vi "G#Debugger_AddObjectToTree.vi"(0 "Front Panel":refnum<vi>, 1 "Tree":refnum<vi>, 2 "Elements":T1[](array[typedef]), 5 "error in (no error)":errorcluster) -> (19 "error out":errorcluster)   [LabVIEW 2017, in "G#Debugger.lvlib"]
uses:
  G#Debugger.lvlib
  G#Debugger_TreeElement.ctl
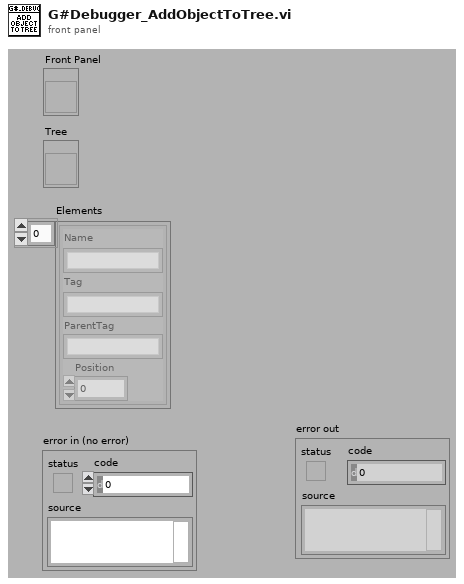
[diagram p1: front panel]
types:
  T1 = typedef "G#Debugger.lvlib/G#Debugger_TreeElement.ctl" = cluster{"Name":string, "Tag":string, "ParentTag":string, "Position":i32}
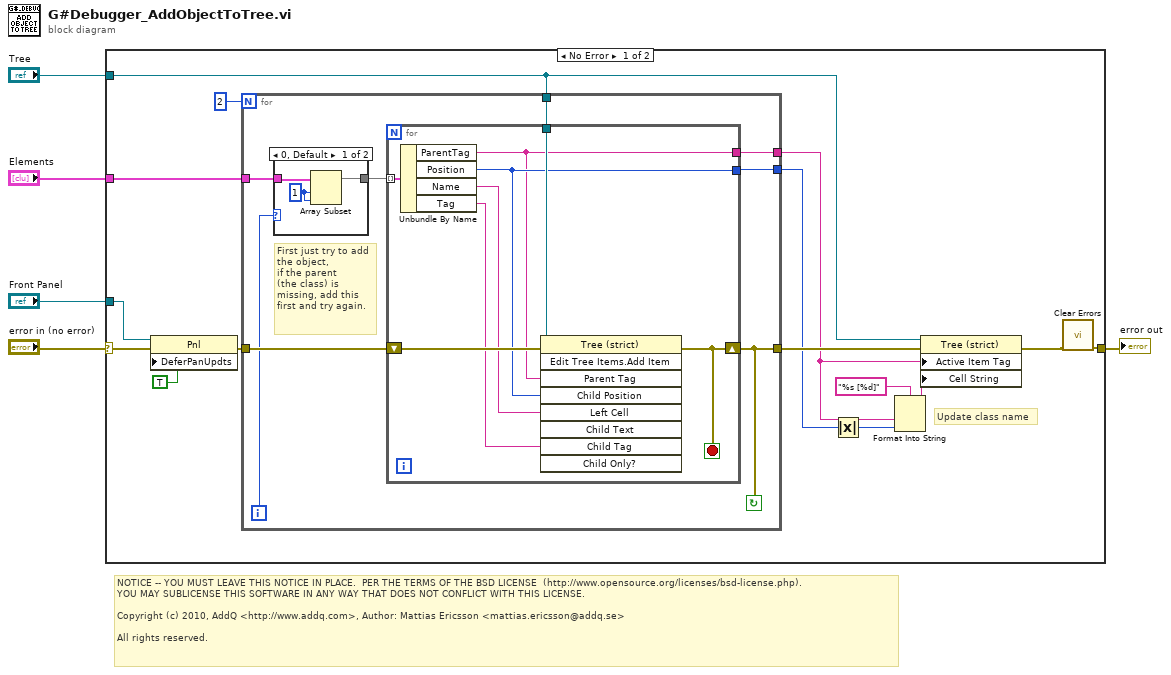
[diagram p0: block diagram]
diagram:
  # "NOTICE -- YOU MUST LEAVE THIS NOTICE IN PLACE.  PER THE TERMS OF THE BSD LICENSE  (http://www.opensource.org/licenses/bsd-license.php).\nYOU MAY SUBLICENSE THIS SOFTWARE IN ANY WAY THAT DOES NOT CONFLICT WITH THIS LICENSE.\n\nCopyright (c) 2010, AddQ <http://www.addq.com>, Author: Mattias Ericsson <mattias.ericsson@addq.se>\n\nAll rights reserved."
  n1 = case shown="No Error" "error in (no error)" {
    selector: "error in (no error)" -> [w6 w41]
    tunnel: [w8 w41] -> w4
    tunnel: "Tree" -> [w19 _]
    tunnel: "Elements" -> [w13 _]
    tunnel: "Front Panel" -> [w7 _]
    frame No Error {
      # "Update class name"
      n2 = property class="Pnl"(reference=w7, error in=w6, "DeferPanUpdts"=TRUE ("Defer Panel Updates")) -> (error out=w11:errorcluster)  [unwired: 1 out]
      n3 = for {
        N: 2 -> [_]
        tunnel: w11 -> [w28]
        tunnel: [w24] -> w20
        tunnel: w19 -> [w27]
        tunnel: [w26] -> w18
        tunnel: [w25] -> w15
        tunnel: w13 -> [w22]
        i -> [w23]
        stop <- w24 continue-if-true
        # "First just try to add\nthe object,\nif the parent\n(the class) is\nmissing, add this\nfirst and try again."
        n4 = case shown="0, Default" w23 {
          tunnel: w22 -> [w31 w32]
          tunnel: [w30 w32] -> w21
          frame 0, Default {
            w29 = 1 ("index")
            n5 = Array Subset(array=w31, index=w29, length=w29) -> (w30:T1[])
          }
          frame 1 {
          }
        }
        n6 = for {
          tunnel: w27 -> [w40]
          shift-right: [w33] -> w24
          shift-left: w28 -> [w39]
          tunnel: w21 -> [w38] mode=indexing
          tunnel: [w35] -> w25
          tunnel: [w34] -> w26
          stop <- w33 stop-if-true
          n7 = Unbundle By Name(w38) -> ("ParentTag"=w34:string, "Position"=w35:i32, "Name"=w37:string, "Tag"=w36:string)
          n8 = invoke class="Tree (strict)" method="Edit Tree Items.Add Item"(reference=w40, error in=w39, "Parent Tag"=w34, "Child Position"=w35, "Left Cell"=w37, "Child Tag"=w36) -> (error out=w33:errorcluster)  [unwired: 3 in, 8 out]
        }
      }
      n9 = Absolute Value(x=w15) -> (abs(x)=w12:i32)
      n10 = Format Into String(format string="%s [%d]", w18, w12) -> (resulting string=w16:string)  [unwired: 2 in, 1 out]
      n11 = property class="Tree (strict)"(reference=w19, error in=w20, "Active Item Tag"=w18, "Cell String"=w16) -> (error out=w9:errorcluster)  [unwired: 1 out]
      n12 = call <vilib>:"Clear Errors.vi"("error in (no error)"=w9) -> ("error out"=w8:errorcluster)  [unwired: 5 in, 1 out]
    }
    frame Error {
    }
  }
  "error out" <- w4
